vi "TCP-String Ack.vi"(0 "connection ID":refnum<k5>, 11 "error in (no error)":errorcluster) -> (4 "connection ID out":refnum<k5>, 15 "error out":errorcluster)   [LabVIEW 2020]
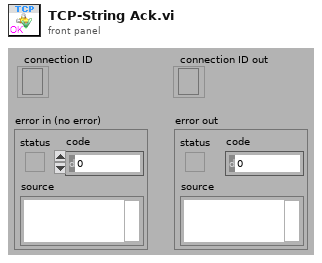
[diagram p1: front panel]
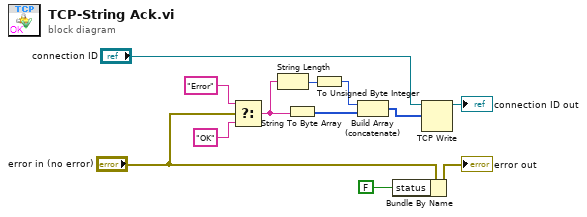
[diagram p0: block diagram]
diagram:
  n1 = Select(t="Error", s="error in (no error)", f="OK") -> (s? t:f=w4:string)
  n2 = String Length(string=w4) -> (length=w3:i32)
  n3 = String To Byte Array(string=w4) -> (unsigned byte array=w6:u8[])
  n4 = To Unsigned Byte Integer(number=w3) -> (unsigned 8bit integer=w2:u8)
  n5 = Build Array (concatenate)(w2, w6) -> (w5:u8[])
  n6 = Bundle By Name(cluster="error in (no error)", "status"=FALSE) -> (→"error out":errorcluster)
  n7 = TCP Write(connection ID="connection ID", data in=w5) -> (connection ID out=→"connection ID out":refnum<k5>)  [unwired: 2 in, 2 out]
